vi "UHR-Fleezers Control (host) - 12.0.vi"() -> ()   [LabVIEW 2012] (continued)
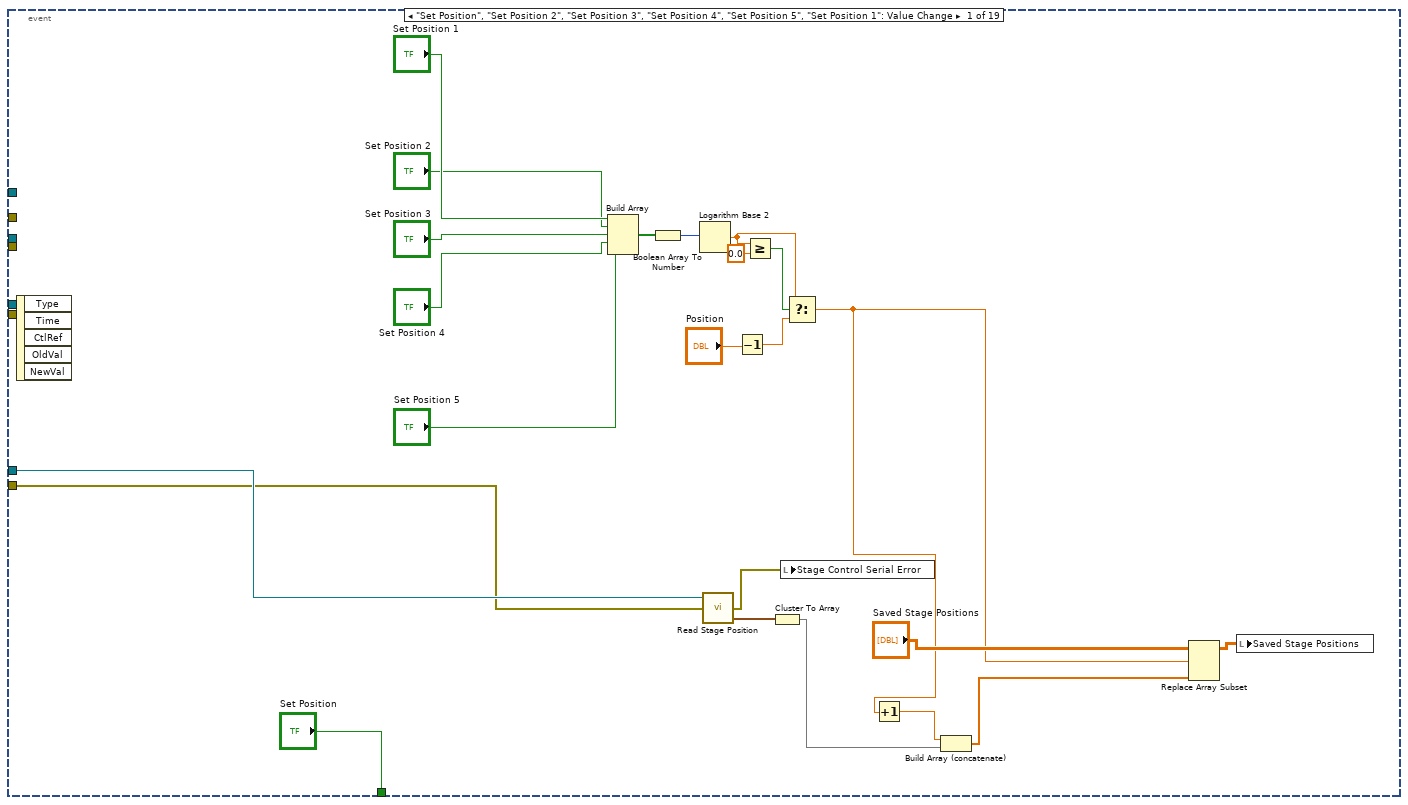
[diagram p3: hidden frame]
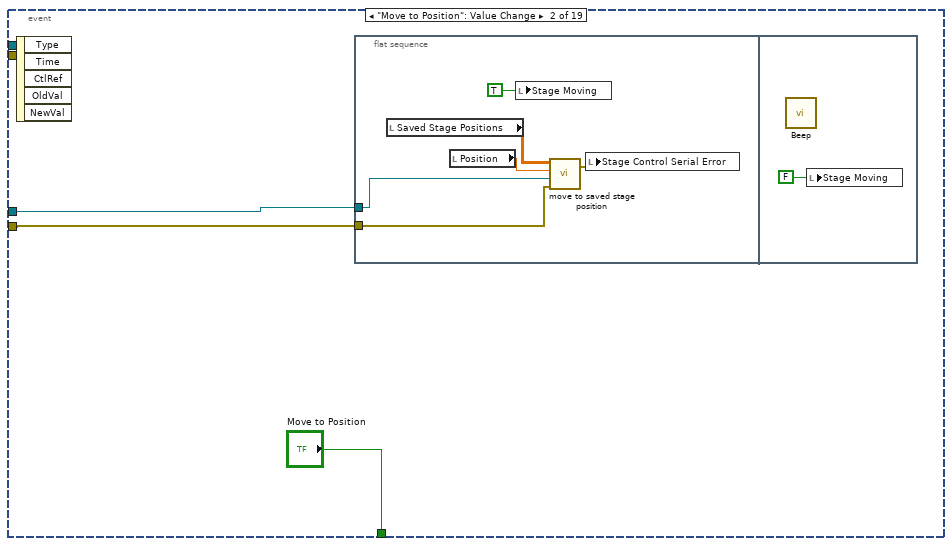
[diagram p4: hidden frame]
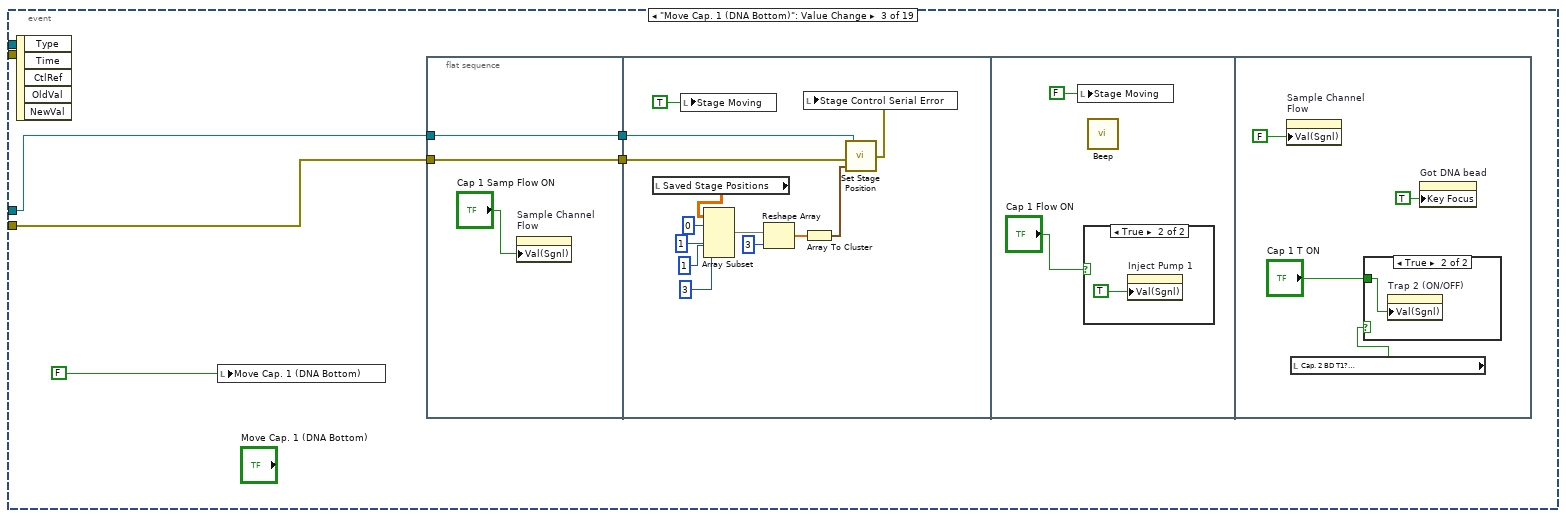
[diagram p5: hidden frame]
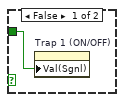
[diagram p7: hidden frame]
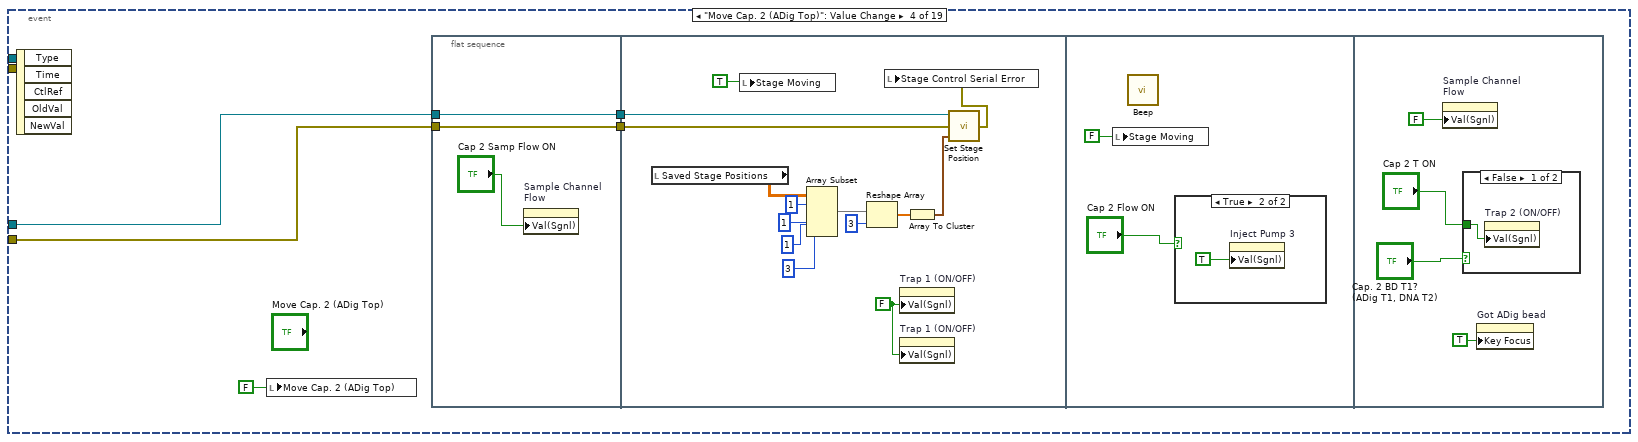
[diagram p8: hidden frame]
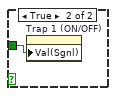
[diagram p10: hidden frame]
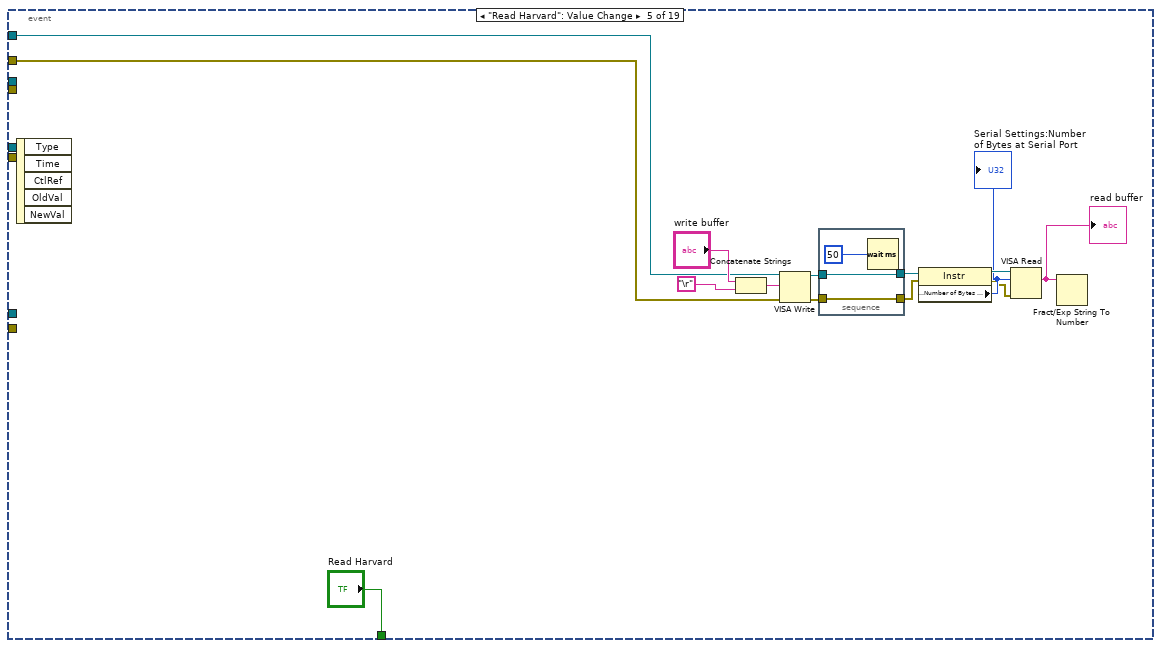
[diagram p11: hidden frame]
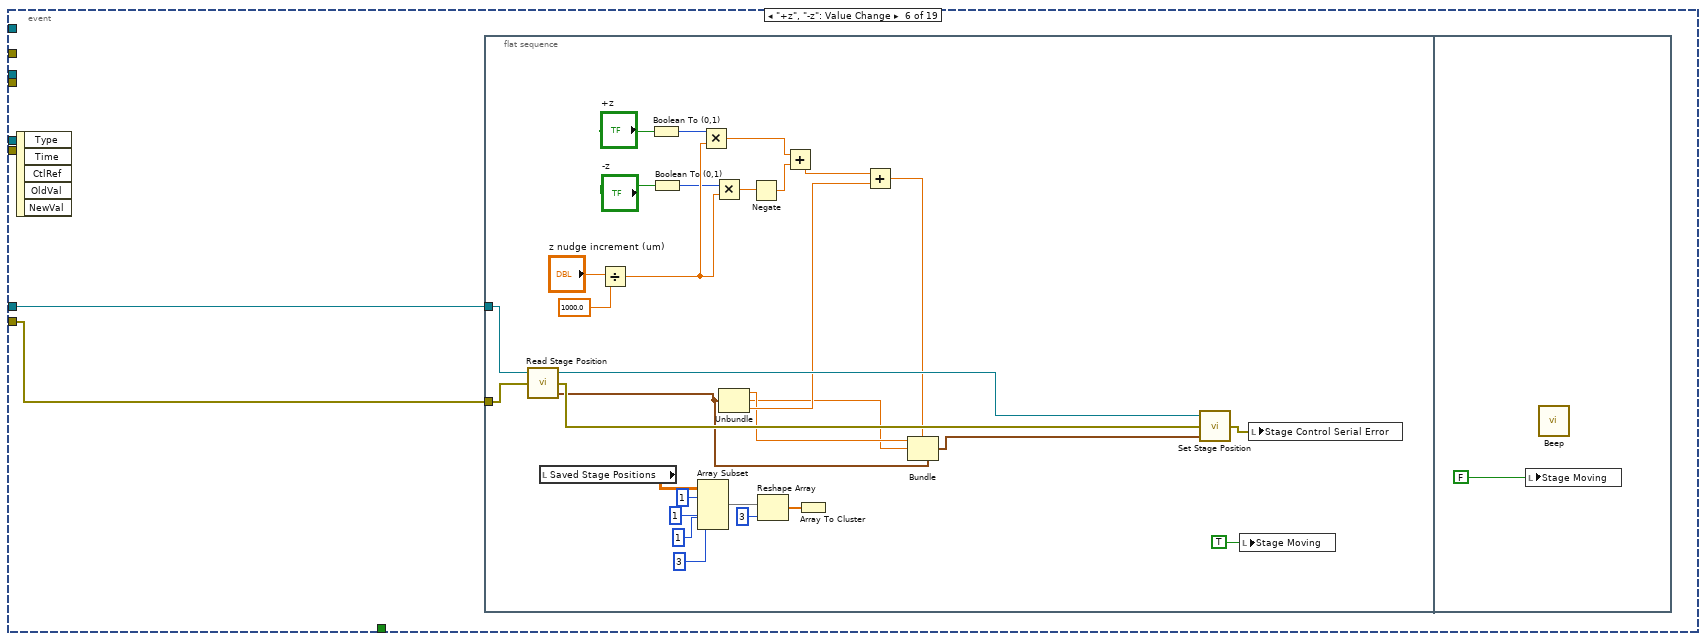
[diagram p12: hidden frame]
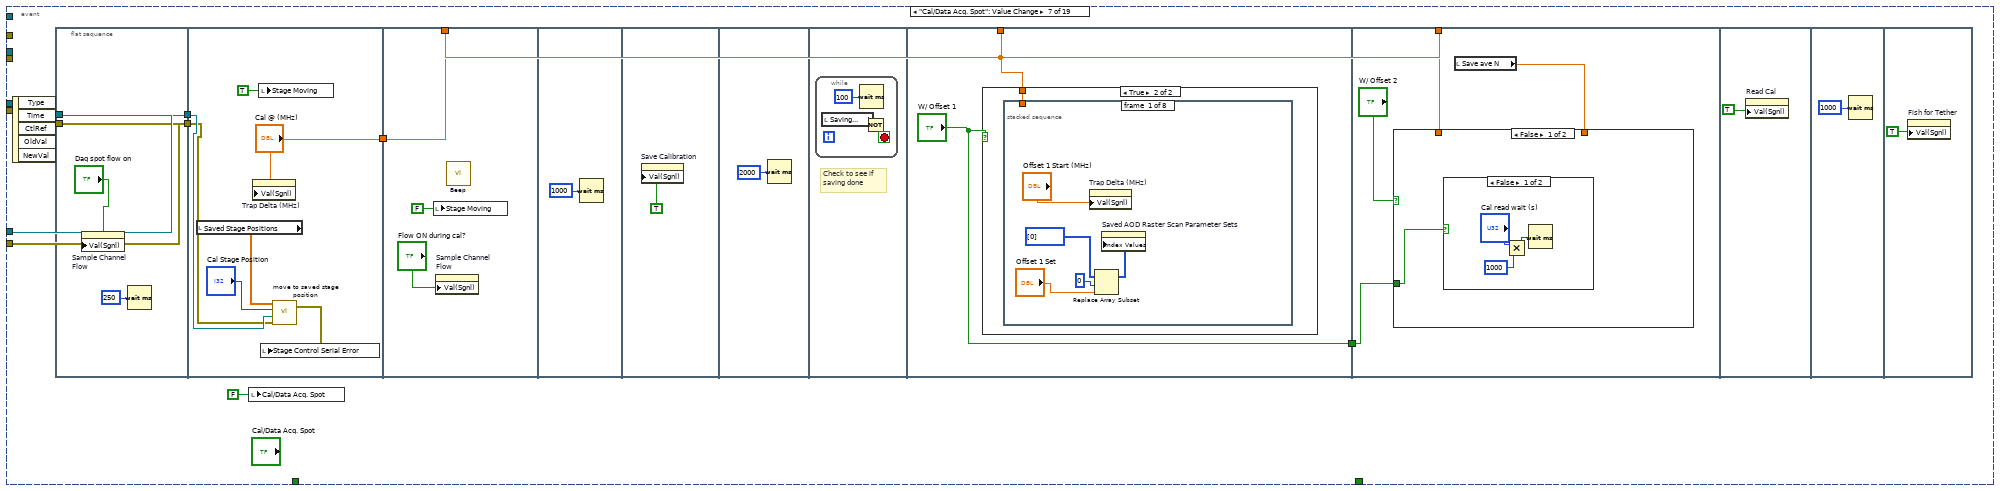
[diagram p13: hidden frame]
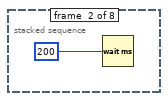
[diagram p15: hidden frame]
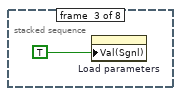
[diagram p16: hidden frame]
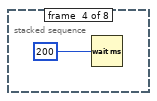
[diagram p17: hidden frame]
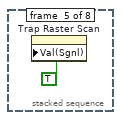
[diagram p18: hidden frame]
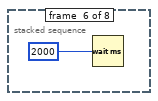
[diagram p19: hidden frame]
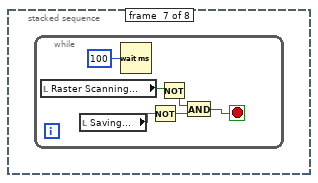
[diagram p20: hidden frame]
                                n2883 = local read "Confocal Y 1 (V)"() -> (w4648:dbl)
                                n2884 = local read "Confocal X 1 (V)"() -> (w4647:dbl)
                                n2885 = property on="AO2" class="Slide (strict)"("Val(Sgnl)"=w4647) -> ()  [unwired: 2 in, 2 out]
                                n2886 = property on="AO1" class="Slide (strict)"("Val(Sgnl)"=w4648) -> ()  [unwired: 2 in, 2 out]
                                }
                                }
                                }
                                }
                                }
                                }
                                }
                                }
                                }
                                }
                                n2887 = local read "Time (s)"() -> (w4585:dbl)
                                n2888 = Subtract(x=w4586, y=w4585) -> (x-y=w4597:dbl)
                                n2889 = Number To Decimal String(number=w4597, width (-)=i16 0) -> (decimal integer string=w4595:string)
                                n2890 = Concatenate Strings(w4595, " s fluorescence event") -> (w4592:string)
                                n2891 = local read "Messages"() -> (w4593:string)
                                n2892 = local write "Duration (s)"(w4597) -> ()
                                n2893 = call "Update messages.vi"("Message to add"=w4592, "Old message string"=w4593) -> ("New message string"=w4591:string)
                                n2894 = local write "Messages"(w4591) -> ()
                                n2895 = call <vilib>:"Beep.vi"() -> ()  [unwired: 12 in]
                                n2896 = local write "Reset Force"(FALSE ("Force Reset")) -> ()
                                n2897 = local write "Fl. High"(TRUE ("Fl. High")) -> ()
                                n2898 = local write "Waiting"(TRUE ("Waiting")) -> ()
                                }
                                }
                                n2899 = node-c288() -> ()  [unwired: 1 in, 1 out]
                                }
                                n2900 = node-c288(w4564) -> ()  [unwired: 1 out]
                                }
                              }
                            }
                          }
                          n2901 = local read "Trap Delta (MHz)"() -> (w4476:dbl)
                          n2902 = local read "Trap Pos FB SP"() -> (w4474:fxp<+/-,16,1>)
                        }
                      }
                    }
                    frame True {
                      n2903 = flat-sequence {
                        tunnel: w4661 -> [w4671]
                        tunnel: [w4671] -> w4665
                        tunnel: w4664 -> [w4670]
                        tunnel: [w4670] -> w4663
                        tunnel: [w4669] -> w4662
                        tunnel: w4660 -> [w4668]
                        tunnel: [w4667] -> w4659
                        tunnel: w4656 -> [w4666]
                        tunnel: [w4666] -> w4655
                        tunnel: w4665 -> [w4741]
                        tunnel: w4663 -> [w4740]
                        tunnel: w4662 -> [w4739]
                        tunnel: w4659 -> [w4738]
                        tunnel: w4655 -> [w4737]
                        tunnel: [w4738] -> w4658
                        frame #0 {
                          n2904 = call <vilib>:"Beep.vi"() -> ()  [unwired: 3 in, 9 out]
                          n2905 = local write "Waiting"(FALSE ("Waiting")) -> ()
                          n2906 = Increment(x=w4668) -> (x+1=w4667:u8)
                          n2907 = case shown="\"Yank\"" w4670 {
                            tunnel: w4667 -> [_ _ w4677]
                            frame "Image" {
                              n2908 = property on="Confocal Image" class="Bool (strict)"("Val(Sgnl)"=TRUE ("Value (Signaling)")) -> ()  [unwired: 2 in, 2 out]
                            }
                            frame "Alarm", Default {
                            }
                            frame "Yank" {
                              n2909 = flat-sequence {
                                tunnel: w4677 -> [w4680]
                                tunnel: [w4679] -> w4676
                                tunnel: ["N Array El"] -> w4675
                                tunnel: w4676 -> [w4694]
                                tunnel: w4675 -> [w4690]
                                frame #0 {
                                n2910 = Multiply(x="Yank Delay (s)", y=1000.0) -> (x*y=w4683:dbl)
                                n2911 = Quotient & Remainder(x=w4680, y="N Array El") -> (x-y*floor(x/y)=w4679:u8)  [unwired: 1 out]
                                n2912 = Wait (ms)(milliseconds to wait=w4683) -> ()  [unwired: 1 out]
                                }
                                frame #1 {
                                n2913 = Random Number (0-1)() -> (number: 0 to 1=w4691:dbl)
                                n2914 = Multiply(x=w4690, y=w4691) -> (x*y=w4689:dbl)
                                n2915 = Round Toward -Infinity(1:w4689) -> (0:w4688:dbl)
                                n2916 = Select(t=w4688, s="Random Choice", f=w4694) -> (s? t:f=w4692:dbl)
                                n2917 = Select(t="Yank to Trap Delta (MHz)", s="Yank to which?", f="Yank to SP") -> (s? t:f=w4685:dbl[])
                                n2918 = Index Array(array=w4685, index=w4692) -> (element=w4695:dbl)
                                n2919 = case shown="False" "Yank to which?" {
                                tunnel: w4695 -> [w4696 w4722]
                                frame False {
                                n2920 = flat-sequence {
                                tunnel: w4696 -> [w4697]
                                frame #0 {
                                n2921 = property on="Trap Pos FB SP" class="DigNum (strict)"("Val(Sgnl)"=w4697) -> ()  [unwired: 2 in, 2 out]
                                }
                                frame #1 {
                                n2922 = Wait (ms)(milliseconds to wait=u32 700) -> ()  [unwired: 1 out]
                                }
                                frame #2 {
                                n2923 = local read "Action (%)"() -> (w4702:dbl)
                                n2924 = Absolute Value(x=w4702) -> (abs(x)=w4701:dbl)
                                n2925 = Greater?(x=w4701, y=70.0) -> (0:w4699:bool)
                                n2926 = property on="Remove Action Offset" class="Bool (strict)"("Val(Sgnl)"=w4699) -> ()  [unwired: 2 in, 2 out]
                                }
                                frame #3 {
                                n2927 = for {
                                N: 4 -> [_]
                                n2928 = flat-sequence {
                                frame #0 {
                                n2929 = Wait (ms)(milliseconds to wait=u32 500) -> ()  [unwired: 1 out]
                                }
                                frame #1 {
                                n2930 = local read "Action (%)"() -> (w4708:dbl)
                                n2931 = Absolute Value(x=w4708) -> (abs(x)=w4707:dbl)
                                n2932 = Greater?(x=w4707, y=70.0) -> (0:w4705:bool)
                                n2933 = property on="Remove Action Offset" class="Bool (strict)"("Val(Sgnl)"=w4705) -> ()  [unwired: 2 in, 2 out]
                                }
                                }
                                }
                                }
                                frame #4 {
                                n2934 = local read "Shift confocal"() -> (w4712:bool)
                                n2935 = local read "Mean"() -> (w4715:dbl)
                                n2936 = Greater?(x=w4715, y=11.0) -> (0:w4711:bool)
                                n2937 = Not(x=w4711) -> (.not. x?=w4710:bool)
                                n2938 = And(x=w4710, y=w4712) -> (x .and. y?=w4709:bool)
                                n2939 = And(x=w4711, y=w4712) -> (x .and. y?=w4713:bool)
                                n2940 = case shown="True" w4713 {
                                frame False {
                                }
                                frame True {
                                n2941 = local read "Confocal X 2 (V)"() -> (w4718:dbl)
                                n2942 = local read "Confocal Y 2 (V)"() -> (w4719:dbl)
                                n2943 = property on="AO2" class="Slide (strict)"("Val(Sgnl)"=w4718) -> ()  [unwired: 2 in, 2 out]
                                n2944 = property on="AO1" class="Slide (strict)"("Val(Sgnl)"=w4719) -> ()  [unwired: 2 in, 2 out]
                                }
                                }
                                n2945 = case shown="True" w4709 {
                                frame False {
                                }
                                frame True {
                                n2946 = local read "Confocal X 1 (V)"() -> (w4716:dbl)
                                n2947 = local read "Confocal Y 1 (V)"() -> (w4717:dbl)
                                n2948 = property on="AO1" class="Slide (strict)"("Val(Sgnl)"=w4717) -> ()  [unwired: 2 in, 2 out]
                                n2949 = property on="AO2" class="Slide (strict)"("Val(Sgnl)"=w4716) -> ()  [unwired: 2 in, 2 out]
                                }
                                }
                                }
                                frame #5 {
                                n2950 = Wait (ms)(milliseconds to wait=u32 1500) -> ()  [unwired: 1 out]
                                }
                                frame #6 {
                                n2951 = property on="Rem fb disp offset" class="Bool (strict)"("Val(Sgnl)"=TRUE ("Value (Signaling)")) -> ()  [unwired: 2 in, 2 out]
                                }
                                }
                                }
                                frame True {
                                n2952 = flat-sequence {
                                tunnel: w4722 -> [w4723]
                                frame #0 {
                                n2953 = property on="Trap Delta (MHz)" class="DigNum (strict)"("Val(Sgnl)"=w4723) -> ()  [unwired: 2 in, 2 out]
                                }
                                frame #1 {
                                n2954 = Wait (ms)(milliseconds to wait=u32 500) -> ()  [unwired: 1 out]
                                }
                                frame #2 {
                                n2955 = local read "Shift confocal"() -> (w4727:bool)
                                n2956 = local read "Mean"() -> (w4725:dbl)
                                n2957 = Greater?(x=w4725, y=11.0) -> (0:w4728:bool)
                                n2958 = Not(x=w4728) -> (.not. x?=w4729:bool)
                                n2959 = And(x=w4729, y=w4727) -> (x .and. y?=w4731:bool)
                                n2960 = And(x=w4728, y=w4727) -> (x .and. y?=w4730:bool)
                                n2961 = case shown="True" w4730 {
                                frame False {
                                }
                                frame True {
                                n2962 = local read "Confocal Y 2 (V)"() -> (w4735:dbl)
                                n2963 = local read "Confocal X 2 (V)"() -> (w4734:dbl)
                                n2964 = property on="AO1" class="Slide (strict)"("Val(Sgnl)"=w4735) -> ()  [unwired: 2 in, 2 out]
                                n2965 = property on="AO2" class="Slide (strict)"("Val(Sgnl)"=w4734) -> ()  [unwired: 2 in, 2 out]
                                }
                                }
                                n2966 = case shown="True" w4731 {
                                frame False {
                                }
                                frame True {
                                n2967 = local read "Confocal X 1 (V)"() -> (w4732:dbl)
                                n2968 = local read "Confocal Y 1 (V)"() -> (w4733:dbl)
                                n2969 = property on="AO2" class="Slide (strict)"("Val(Sgnl)"=w4732) -> ()  [unwired: 2 in, 2 out]
                                n2970 = property on="AO1" class="Slide (strict)"("Val(Sgnl)"=w4733) -> ()  [unwired: 2 in, 2 out]
                                }
                                }
                                }
                                }
                                }
                                }
                                }
                              }
                            }
                          }
                          n2971 = local read "Time (s)"() -> (w4669:dbl)
                          "Fl. High" <- TRUE ("Yanking")
                        }
                        frame #1 {
                          n2972 = local read "Auto F Reset"() -> (w4736:bool)
                          n2973 = case shown="True" w4736 {
                            tunnel: w4741 -> [_ w4745]
                            tunnel: w4740 -> [_ w4744]
                            tunnel: w4739 -> [_ w4743]
                            tunnel: w4737 -> [_ w4742]
                            frame False {
                            }
                            frame True {
                              n2974 = node-c288() -> (w4747:T21)  [unwired: 4 out]
                              n2975 = timed-loop {
                                timing: w4747 -> [_]
                                timing-out: [_] -> w4746
                                tunnel: w4745 -> [w4765]
                                tunnel: w4744 -> [w4764]
                                tunnel: w4743 -> [w4763]
                                tunnel: w4742 -> [w4762]
                                stop <- w4748 stop-if-true
                                n2976 = node-c288() -> ()  [unwired: 2 out]
                                n2977 = local read "Fl. Delta Thresh. (kHz)"() -> (w4756:dbl)
                                n2978 = local read "Fl. Triggered..."() -> (w4761:bool)
                                n2979 = local read "Delta Fl. 1"() -> (w4752:dbl)
                                n2980 = local read "Delta Fl. 2"() -> (w4750:dbl)
                                n2981 = local read "Stop All"() -> (w4759:bool)
                                n2982 = local read "APD to Watch"() -> (w4751:bool)
                                n2983 = Select(t=w4752, s=w4751, f=w4750) -> (s? t:f=w4749:dbl)
                                n2984 = Not(x=w4761) -> (.not. x?=w4760:bool)
                                n2985 = Multiply(x=w4756, y=1000.0) -> (x*y=w4755:dbl)
                                n2986 = Negate(x=w4755) -> (-x=w4754:dbl)
                                n2987 = Less?(x=w4749, y=w4754) -> (x < y?=w4758:bool)
                                n2988 = Compound Arithmetic op=OR(w4758, w4759, w4760, "Reset Force") -> (w4748:bool)
                                n2989 = case shown="True" w4748 {
                                tunnel: w4765 -> [_ w4780]
                                tunnel: w4764 -> [_ w4779]
                                tunnel: w4763 -> [_ w4769]
                                tunnel: w4762 -> [_ w4771]
                                frame False {
                                }
                                frame True {
                                n2990 = local read "Time (s)"() -> (w4770:dbl)
                                n2991 = case shown="\"Yank\"" w4779 {
                                tunnel: w4780 -> [_ w4783]
                                tunnel: w4771 -> [_ w4781]
                                frame "Image", Default {
                                }
                                frame "Yank" {
                                n2992 = flat-sequence {
                                tunnel: [w4789] -> w4784
                                tunnel: w4783 -> [w4789]
                                tunnel: [w4785] -> w4782
                                tunnel: w4781 -> [w4785]
                                tunnel: w4784 -> [w4792]
                                tunnel: w4782 -> [w4790]
                                frame #0 {
                                n2993 = local read "Yank Delay (s)"() -> (w4788:dbl)
                                n2994 = Multiply(x=w4788, y=1000.0) -> (x*y=w4786:dbl)
                                n2995 = Wait (ms)(milliseconds to wait=w4786) -> ()  [unwired: 1 out]
                                }
                                frame #1 {
                                n2996 = local read "Yank to which?"() -> (w4791:bool)
                                n2997 = case shown="False" w4791 {
                                tunnel: w4792 -> [_ w4819]
                                tunnel: w4790 -> [w4793 _]
                                frame False {
                                n2998 = flat-sequence {
                                tunnel: w4793 -> [w4794]
                                frame #0 {
                                n2999 = property on="Trap Pos FB SP" class="DigNum (strict)"("Val(Sgnl)"=w4794) -> ()  [unwired: 2 in, 2 out]
                                }
                                frame #1 {
                                n3000 = Wait (ms)(milliseconds to wait=u32 700) -> ()  [unwired: 1 out]
                                }
                                frame #2 {
                                n3001 = local read "Action (%)"() -> (w4799:dbl)
                                n3002 = Absolute Value(x=w4799) -> (abs(x)=w4798:dbl)
                                n3003 = Greater?(x=w4798, y=70.0) -> (0:w4796:bool)
                                n3004 = property on="Remove Action Offset" class="Bool (strict)"("Val(Sgnl)"=w4796) -> ()  [unwired: 2 in, 2 out]
                                }
                                frame #3 {
                                n3005 = for {
                                N: 4 -> [_]
                                n3006 = flat-sequence {
                                frame #0 {
                                n3007 = Wait (ms)(milliseconds to wait=u32 500) -> ()  [unwired: 1 out]
                                }
                                frame #1 {
                                n3008 = local read "Action (%)"() -> (w4805:dbl)
                                n3009 = Absolute Value(x=w4805) -> (abs(x)=w4804:dbl)
                                n3010 = Greater?(x=w4804, y=70.0) -> (0:w4802:bool)
                                n3011 = property on="Remove Action Offset" class="Bool (strict)"("Val(Sgnl)"=w4802) -> ()  [unwired: 2 in, 2 out]
                                }
                                }
                                }
                                }
                                frame #4 {
                                n3012 = local read "Shift confocal"() -> (w4810:bool)
                                n3013 = local read "Mean"() -> (w4812:dbl)
                                n3014 = Greater?(x=w4812, y=11.0) -> (0:w4809:bool)
                                n3015 = Not(x=w4809) -> (.not. x?=w4808:bool)
                                n3016 = And(x=w4809, y=w4810) -> (x .and. y?=w4807:bool)
                                n3017 = And(x=w4808, y=w4810) -> (x .and. y?=w4806:bool)
                                n3018 = case shown="True" w4807 {
                                frame False {
                                }
                                frame True {
                                n3019 = local read "Confocal Y 2 (V)"() -> (w4816:dbl)
                                n3020 = local read "Confocal X 2 (V)"() -> (w4815:dbl)
                                n3021 = property on="AO2" class="Slide (strict)"("Val(Sgnl)"=w4815) -> ()  [unwired: 2 in, 2 out]
                                n3022 = property on="AO1" class="Slide (strict)"("Val(Sgnl)"=w4816) -> ()  [unwired: 2 in, 2 out]
                                }
                                }
                                n3023 = case shown="True" w4806 {
                                frame False {
                                }
                                frame True {
                                n3024 = local read "Confocal X 1 (V)"() -> (w4813:dbl)
                                n3025 = local read "Confocal Y 1 (V)"() -> (w4814:dbl)
                                n3026 = property on="AO1" class="Slide (strict)"("Val(Sgnl)"=w4814) -> ()  [unwired: 2 in, 2 out]
                                n3027 = property on="AO2" class="Slide (strict)"("Val(Sgnl)"=w4813) -> ()  [unwired: 2 in, 2 out]
                                }
                                }
                                }
                                frame #5 {
                                n3028 = Wait (ms)(milliseconds to wait=u32 1500) -> ()  [unwired: 1 out]
                                }
                                frame #6 {
                                n3029 = property on="Rem fb disp offset" class="Bool (strict)"("Val(Sgnl)"=TRUE ("Value (Signaling)")) -> ()  [unwired: 2 in, 2 out]
                                }
                                }
                                }
                                frame True {
                                n3030 = flat-sequence {
                                tunnel: w4819 -> [w4820]
                                frame #0 {
                                n3031 = property on="Trap Delta (MHz)" class="DigNum (strict)"("Val(Sgnl)"=w4820) -> ()  [unwired: 2 in, 2 out]
                                }
                                frame #1 {
                                n3032 = Wait (ms)(milliseconds to wait=u32 500) -> ()  [unwired: 1 out]
                                }
                                frame #2 {
                                n3033 = local read "Shift confocal"() -> (w4826:bool)
                                n3034 = local read "Mean"() -> (w4828:dbl)
                                n3035 = Greater?(x=w4828, y=11.0) -> (0:w4825:bool)
                                n3036 = Not(x=w4825) -> (.not. x?=w4824:bool)
                                n3037 = And(x=w4825, y=w4826) -> (x .and. y?=w4823:bool)
                                n3038 = And(x=w4824, y=w4826) -> (x .and. y?=w4822:bool)
                                n3039 = case shown="True" w4823 {
                                frame False {
                                }
                                frame True {
                                n3040 = local read "Confocal Y 2 (V)"() -> (w4832:dbl)
                                n3041 = local read "Confocal X 2 (V)"() -> (w4831:dbl)
                                n3042 = property on="AO2" class="Slide (strict)"("Val(Sgnl)"=w4831) -> ()  [unwired: 2 in, 2 out]
                                n3043 = property on="AO1" class="Slide (strict)"("Val(Sgnl)"=w4832) -> ()  [unwired: 2 in, 2 out]
                                }
                                }
                                n3044 = case shown="True" w4822 {
                                frame False {
                                }
                                frame True {
                                n3045 = local read "Confocal Y 1 (V)"() -> (w4830:dbl)
                                n3046 = local read "Confocal X 1 (V)"() -> (w4829:dbl)
                                n3047 = property on="AO2" class="Slide (strict)"("Val(Sgnl)"=w4829) -> ()  [unwired: 2 in, 2 out]
                                n3048 = property on="AO1" class="Slide (strict)"("Val(Sgnl)"=w4830) -> ()  [unwired: 2 in, 2 out]
                                }
                                }
                                }
                                }
                                }
                                }
                                }
                                }
                                }
                                }
                                n3049 = local read "Messages"() -> (w4778:string)
                                n3050 = Subtract(x=w4770, y=w4769) -> (x-y=w4776:dbl)
                                "Duration (s)" <- w4776
                                n3051 = Number To Decimal String(number=w4776, width (-)=i16 0) -> (decimal integer string=w4774:string)
                                n3052 = Concatenate Strings(w4774, " s fluorescence event." ("string")) -> (w4772:string)
                                n3053 = call "Update messages.vi"("Message to add"=w4772, "Old message string"=w4778) -> ("New message string"=w4777:string)
                                n3054 = local write "Reset Force"(FALSE ("Reset Force")) -> ()
                                n3055 = local write "Waiting"(TRUE ("Waiting")) -> ()
                                n3056 = local write "Messages"(w4777) -> ()
                                n3057 = local write "Fl. High"(FALSE ("Fl. High")) -> ()
                                n3058 = call <vilib>:"Beep.vi"() -> ()  [unwired: 3 in, 9 out]
                                }
                                }
                                n3059 = node-c288() -> ()  [unwired: 2 out]
                              }
                              n3060 = node-c288(w4746) -> ()  [unwired: 1 out]
                            }
                          }
                        }
                      }
                      n3061 = local read "Trap Delta (MHz)"() -> (w4661:dbl)
                      n3062 = local read "Trap Pos FB SP"() -> (w4656:fxp<+/-,16,1>)
                    }
                  }
                }
                frame #1 {
                  n3063 = local read "Stop All"() -> (w4842:bool)
                  n3064 = local read "Fl. Triggered..."() -> (w4840:bool)
                  n3065 = Not(x=w4840) -> (.not. x?=w4841:bool)
                  n3066 = Or(x=w4841, y=w4842) -> (x .or. y?=w4839:bool)
                }
              }
              n3067 = case shown="True" w4433 {
                frame False {
                }
                frame True {
                  n3068 = local read "Confocal Y 1 (V)"() -> (w4443:dbl)
                  n3069 = local read "Confocal X 1 (V)"() -> (w4442:dbl)
                  n3070 = property on="AO2" class="Slide (strict)"("Val(Sgnl)"=w4442) -> ()  [unwired: 2 in, 2 out]
                  n3071 = property on="AO1" class="Slide (strict)"("Val(Sgnl)"=w4443) -> ()  [unwired: 2 in, 2 out]
                }
              }
              n3072 = case shown="True" w4433 {
                frame False {
                }
                frame True {
                  w4441 = FALSE ("Fl. High")
                  n3073 = local write "Waiting"(w4441) -> ()
                  n3074 = local write "Fl. High"(w4441) -> ()
                }
              }
              n3075 = node-c288() -> ()  [unwired: 2 out]
            }
            n3076 = node-c288(w4431) -> ()  [unwired: 1 out]
          }
        }
      }
      event "Stop All": Value Change {
        n3077 = event-data() -> ()  [unwired: 7 out]
        n3078 = local read "Stop All"() -> (w4847:bool)
      }
    }
    n3079 = node-c288() -> ()  [unwired: 2 out]
  }
  n3080 = node-c288(w96) -> ()  [unwired: 1 out]
  n3081 = node-c288(w98) -> ()  [unwired: 1 out]
  n3082 = node-c288(w83) -> ()  [unwired: 1 out]
  n3083 = property on="Saved trap pos" class="WFGraph (strict)"("Visible"=FALSE) -> ()  [unwired: 2 in, 2 out]
  n3084 = property on="Trap Delta Graph" class="WFGraph (strict)"("Visible"=TRUE) -> ()  [unwired: 2 in, 2 out]
  n3085 = local write "Trap pos"(FALSE ("Trap pos")) -> ()
  n3086 = local write "Offset (nm)"(0.0 ("Offset (nm)")) -> ()
  n3087 = local write "Bead Mean (nm)"(0.0 ("Bead Mean (nm)")) -> ()
  n3088 = disable-structure shown="Disabled" {
    disable-tunnel: w87 -> [w4849 _]
    disable-tunnel: w86 -> [w4848 _]
    frame Disabled {
      n3089 = VISA Close(VISA resource name=w4849, error in (no error)=w4848) -> (error out=w4850:errorcluster)
      n3090 = call <vilib>:"Simple Error Handler.vi"("error in (no error)"=w4850) -> ()  [unwired: 1 in, 8 out]
    }
    frame Enabled {
    }
  }
  n3091 = node-c288(w178) -> ()  [unwired: 1 out]
  n3092 = node-c288(w94) -> ()  [unwired: 1 out]
  n3093 = flat-sequence {
    tunnel: w272 -> [w4854]
    tunnel: w274 -> [w4855]
    tunnel: [w4853] -> w253
    tunnel: [w4852] -> w252
    tunnel: w234 -> [_]
    tunnel: w186 -> [_]
    tunnel: w100 -> [_]
    tunnel: w253 -> [w4856]
    tunnel: w252 -> [w4857]
    frame #0 {
      w4851 = FALSE ("AI to FIFO")
      n3094 = xnode "Read/Write Control"("FPGA VI Reference In"=w4855, "error in"=w4854, "AI to FIFO"=w4851, "APD to FIFO"=w4851) -> ("FPGA VI Reference Out"=w4853:T19, "error out"=w4852:errorcluster)
    }
    frame #1 {
      n3095 = xnode "Close FPGA VI Reference"("FPGA VI Reference In"=w4856, "error in"=w4857) -> ("error out"=→"error out":errorcluster)
    }
  }
